vi "Get Score.vi"(11 "Game Board in":refnum<class "Game Board.lvclass">) -> (2 "Score":u32)   [LabVIEW 2020, in "Game Board.lvclass"]
uses:
  Game Board.lvclass
  Game Board.lvclass/Game Board.ctl
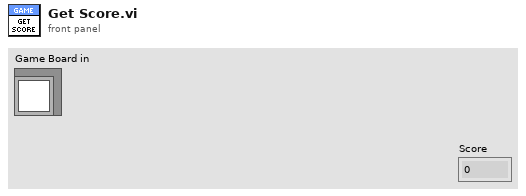
[diagram p1: front panel]
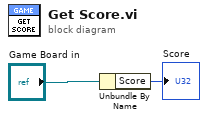
[diagram p0: block diagram]
diagram:
  n1 = Unbundle By Name("Game Board in") -> ("Score"=→"Score":u32)
